vi "AbortEventCreator.vi"(0 "Add Event":bool, 1 "Enable":bool, 2 "P#":dbl, 3 "Event Name":string, 4 "Sensor Select":u16(ring) items=["", "PT1", "PT2", "PT3", "TC1", "TC2", "LP1", "LS1", "LS2"], 5 "H":dbl, 6 "L":dbl, 7 "Remove Event":bool, 8 "SV6":bool, 10 "SV5":bool, 12 "SV4":bool, 14 "SV3":bool, 16 "SV2":bool, 18 "SV1":bool, 20 "SV0":bool) -> (9 "SV6":bool[](array[boolean]), 11 "SV5":bool[](array[boolean]), 13 "SV4":bool[](array[boolean]), 15 "SV3":bool[](array[boolean]), 17 "SV2":bool[](array[boolean]), 19 "SV1":bool[](array[boolean]), 21 "Enable":bool[](array[boolean]), 22 "P#":dbl[](array[numeric]), 23 "Event Name":string[](array[string]), 24 "Sensor Select":u16[](array[ring]) items=["", "PT1", "PT2", "PT3", "TC1", "TC2", "LP1", "LS1", "LS2"], 25 "H":dbl[](array[numeric]), 26 "L":dbl[](array[numeric]), 27 "SV0":bool[](array[boolean]))   [LabVIEW 2021]
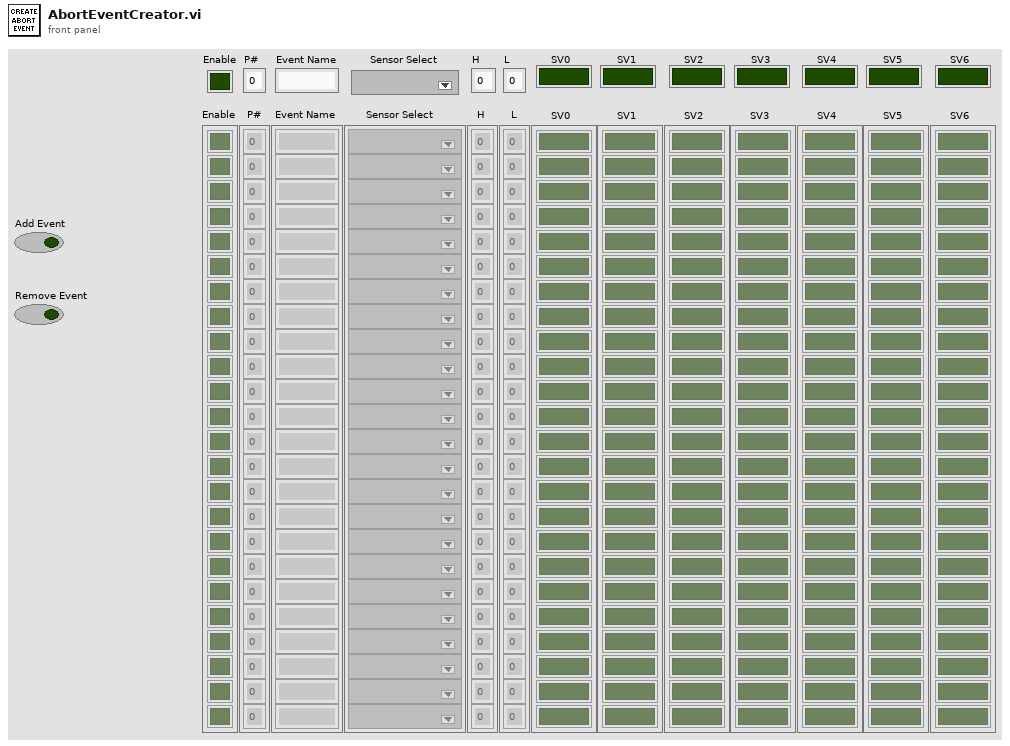
[diagram p1: front panel]
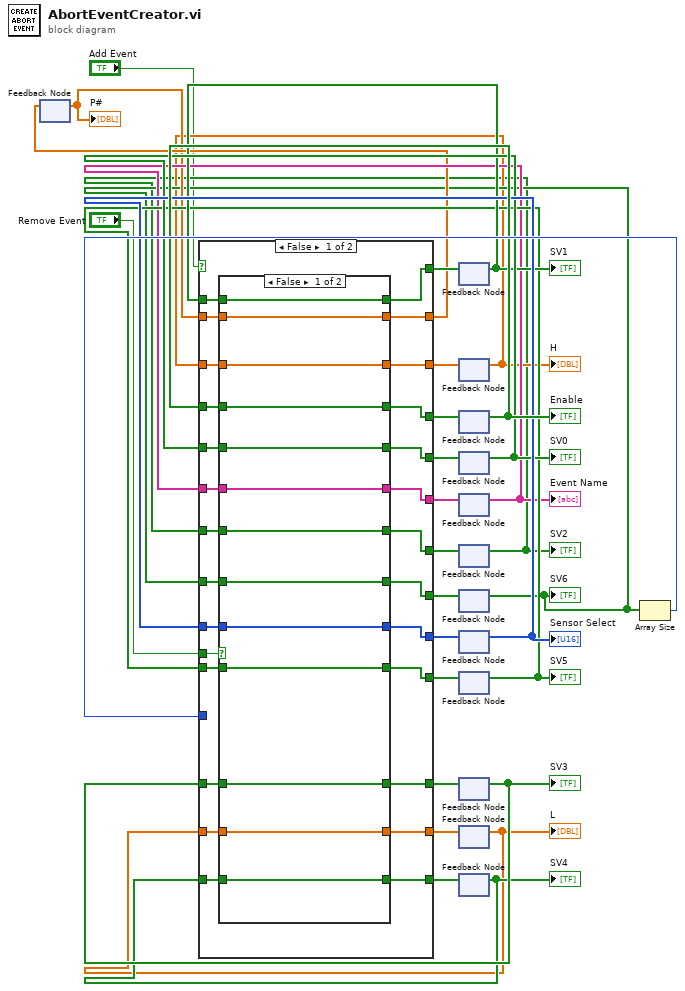
[diagram p0: block diagram]
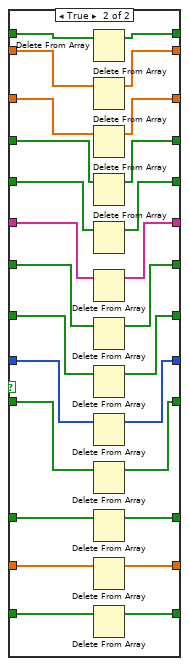
[diagram p2: hidden frame]
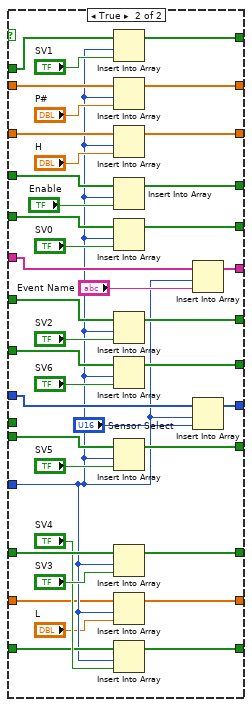
[diagram p3: hidden frame]
diagram:
  n1 = feedback #1() -> (w9:dbl[])  [unwired: 1 in]
  "P#" <- w9
  n2 = feedback #2() -> (w21:bool[])  [unwired: 1 in]
  "SV1" <- w21
  n3 = feedback #3() -> (w6:dbl[])  [unwired: 1 in]
  "H" <- w6
  n4 = feedback #4() -> (w27:bool[])  [unwired: 1 in]
  "Enable" <- w27
  n5 = feedback #5() -> (w23:bool[])  [unwired: 1 in]
  "SV0" <- w23
  n6 = feedback #6() -> (w11:string[])  [unwired: 1 in]
  "Event Name" <- w11
  n7 = feedback #7() -> (w3:bool[])  [unwired: 1 in]
  "SV2" <- w3
  n8 = feedback #8() -> (w8:bool[])  [unwired: 1 in]
  "SV6" <- w8
  n9 = feedback #9() -> (w25:u16[])  [unwired: 1 in]
  "Sensor Select" <- w25
  n10 = feedback #10() -> (w14:bool[])  [unwired: 1 in]
  "SV5" <- w14
  n11 = feedback #11() -> (w18:bool[])  [unwired: 1 in]
  "SV3" <- w18
  n12 = feedback #12() -> (w4:dbl[])  [unwired: 1 in]
  "L" <- w4
  n13 = feedback #13() -> (w16:bool[])  [unwired: 1 in]
  "SV4" <- w16
  n14 = Array Size(array=w8) -> (size(s)=w29:i32)
  n15 = case shown="False" "Add Event" {
    tunnel: w29 -> [_ w100]
    tunnel: [w39 w134] -> w28
    tunnel: w27 -> [w40 w135]
    tunnel: [w44 w132] -> w26
    tunnel: w25 -> [w43 w131]
    tunnel: [w50 w128] -> w24
    tunnel: w23 -> [w49 w127]
    tunnel: [w47 w126] -> w22
    tunnel: w21 -> [w48 w125]
    tunnel: [w56 w123] -> w20
    tunnel: w3 -> [w55 w122]
    tunnel: w18 -> [w53 w120]
    tunnel: [w54 w119] -> w19
    tunnel: w16 -> [w51 w117]
    tunnel: [w52 w116] -> w17
    tunnel: w14 -> [w45 w114]
    tunnel: [w46 w113] -> w15
    tunnel: w8 -> [w42 w112]
    tunnel: [w41 w111] -> w13
    tunnel: w11 -> [w37 w109]
    tunnel: [w38 w108] -> w12
    tunnel: w9 -> [w35 w105]
    tunnel: [w36 w104] -> w10
    tunnel: w6 -> [w31 w102]
    tunnel: [w32 w101] -> w7
    tunnel: w4 -> [w33 w98]
    tunnel: [w34 w97] -> w5
    tunnel: "Remove Event" -> [w30 _]
    frame False {
      n16 = case shown="False" w30 {
        tunnel: [w57 w95] -> w56
        tunnel: w55 -> [w57 w94]
        tunnel: [w59 w93] -> w54
        tunnel: w53 -> [w59 w92]
        tunnel: [w60 w91] -> w52
        tunnel: w51 -> [w60 w90]
        tunnel: [w61 w89] -> w50
        tunnel: w49 -> [w61 w88]
        tunnel: w48 -> [w63 w87]
        tunnel: [w63 w86] -> w47
        tunnel: [w64 w85] -> w46
        tunnel: w45 -> [w64 w84]
        tunnel: [w58 w83] -> w44
        tunnel: w43 -> [w58 w82]
        tunnel: w42 -> [w69 w81]
        tunnel: [w69 w80] -> w41
        tunnel: w40 -> [w68 w79]
        tunnel: [w68 w78] -> w39
        tunnel: [w67 w77] -> w38
        tunnel: w37 -> [w67 w76]
        tunnel: [w66 w75] -> w36
        tunnel: w35 -> [w66 w74]
        tunnel: [w65 w73] -> w34
        tunnel: w33 -> [w65 w72]
        tunnel: [w62 w71] -> w32
        tunnel: w31 -> [w62 w70]
        frame False {
        }
        frame True {
          n17 = Delete From Array(array=w87) -> (array with subset deleted=w86:bool[])  [unwired: 2 in, 1 out]
          n18 = Delete From Array(array=w74) -> (array with subset deleted=w75:dbl[])  [unwired: 2 in, 1 out]
          n19 = Delete From Array(array=w70) -> (array with subset deleted=w71:dbl[])  [unwired: 2 in, 1 out]
          n20 = Delete From Array(array=w79) -> (array with subset deleted=w78:bool[])  [unwired: 2 in, 1 out]
          n21 = Delete From Array(array=w88) -> (array with subset deleted=w89:bool[])  [unwired: 2 in, 1 out]
          n22 = Delete From Array(array=w76) -> (array with subset deleted=w77:string[])  [unwired: 2 in, 1 out]
          n23 = Delete From Array(array=w94) -> (array with subset deleted=w95:bool[])  [unwired: 2 in, 1 out]
          n24 = Delete From Array(array=w81) -> (array with subset deleted=w80:bool[])  [unwired: 2 in, 1 out]
          n25 = Delete From Array(array=w82) -> (array with subset deleted=w83:u16[])  [unwired: 2 in, 1 out]
          n26 = Delete From Array(array=w84) -> (array with subset deleted=w85:bool[])  [unwired: 2 in, 1 out]
          n27 = Delete From Array(array=w92) -> (array with subset deleted=w93:bool[])  [unwired: 2 in, 1 out]
          n28 = Delete From Array(array=w72) -> (array with subset deleted=w73:dbl[])  [unwired: 2 in, 1 out]
          n29 = Delete From Array(array=w90) -> (array with subset deleted=w91:bool[])  [unwired: 2 in, 1 out]
        }
      }
    }
    frame True {
      n30 = Insert Into Array(array=w125, index=w100, new element="SV1") -> (w126:bool[])
      n31 = Insert Into Array(array=w105, index=w100, new element="P#") -> (w104:dbl[])
      n32 = Insert Into Array(array=w102, index=w100, new element="H") -> (w101:dbl[])
      n33 = Insert Into Array(array=w135, index=w100, new element="Enable") -> (w134:bool[])
      n34 = Insert Into Array(array=w127, index=w100, new element="SV0") -> (w128:bool[])
      n35 = Insert Into Array(array=w122, index=w100, new element="SV2") -> (w123:bool[])
      n36 = Insert Into Array(array=w112, index=w100, new element="SV6") -> (w111:bool[])
      n37 = Insert Into Array(array=w114, index=w100, new element="SV5") -> (w113:bool[])
      n38 = Insert Into Array(array=w120, index=w100, new element="SV3") -> (w119:bool[])
      n39 = Insert Into Array(array=w98, index=w100, new element="L") -> (w97:dbl[])
      n40 = Insert Into Array(array=w117, index=w100, new element="SV4") -> (w116:bool[])
      n41 = Insert Into Array(array=w109, index=w100, new element="Event Name") -> (w108:string[])
      n42 = Insert Into Array(array=w131, index=w100, new element="Sensor Select") -> (w132:u16[])
    }
  }
  n43 = feedback-in #1(w10) -> ()
  n44 = feedback-in #2(w22) -> ()
  n45 = feedback-in #3(w7) -> ()
  n46 = feedback-in #4(w28) -> ()
  n47 = feedback-in #5(w24) -> ()
  n48 = feedback-in #6(w12) -> ()
  n49 = feedback-in #7(w20) -> ()
  n50 = feedback-in #8(w13) -> ()
  n51 = feedback-in #9(w26) -> ()
  n52 = feedback-in #10(w15) -> ()
  n53 = feedback-in #11(w19) -> ()
  n54 = feedback-in #12(w5) -> ()
  n55 = feedback-in #13(w17) -> ()
